vi "PSU updated.vi"() -> ()   [LabVIEW 2012]
panel:
  in  "PSU updated":bool
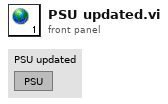
[diagram p1: front panel]
diagram:
